vi "FGV_UE.vi"(7 "State":T1, 8 "Error In":errorcluster) -> (0 "Error Out":errorcluster, 3 "STOP":refnum<user-event>)   [LabVIEW 2017, in "StopUE.lvlib"]
uses:
  StopUE.lvlib
  States_FGV.ctl
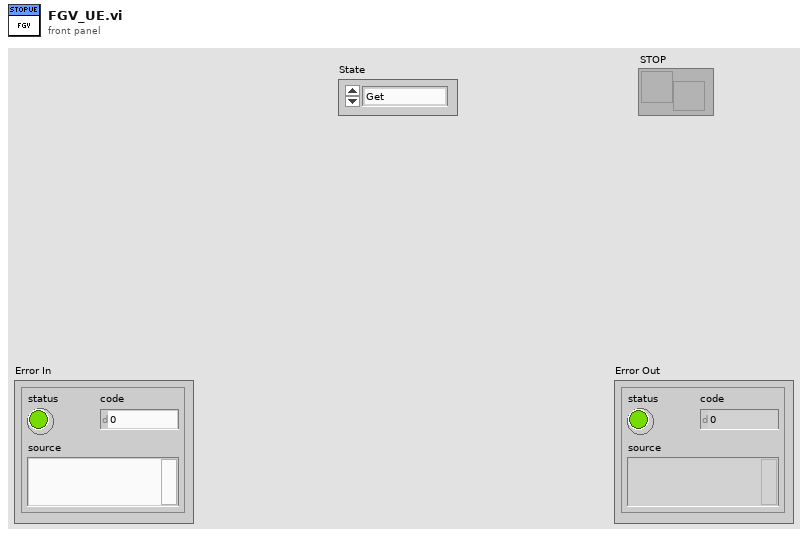
[diagram p1: front panel]
types:
  T1 = typedef "StopUE.lvlib/States_FGV.ctl" = enum16{"Get", "Shutdown", "Initialize"}
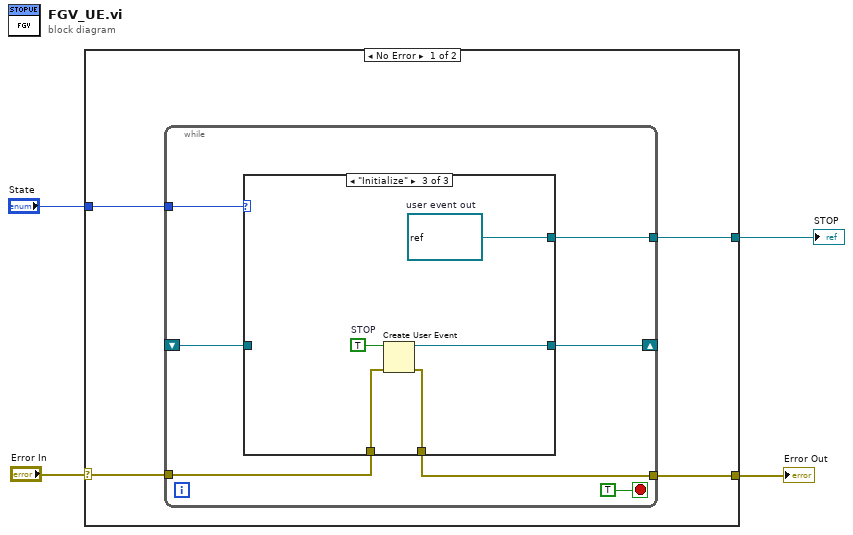
[diagram p0: block diagram]
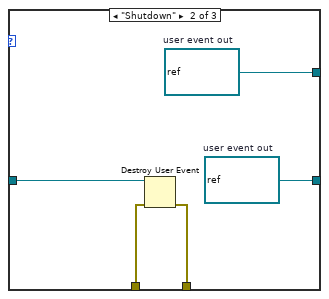
[diagram p3: hidden frame]
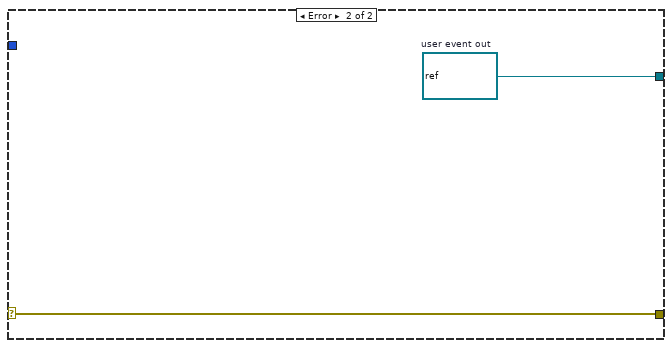
[diagram p4: hidden frame]
diagram:
  n1 = case shown="No Error" "Error In" {
    selector: "Error In" -> [w8 w28]
    tunnel: "State" -> [w7 _]
    tunnel: [w6 w28] -> w2
    tunnel: [w5 w29] -> w1
    frame No Error {
      n2 = while {
        tunnel: w8 -> [w13]
        tunnel: w7 -> [w14]
        tunnel: [w12] -> w6
        shift-right: [w11] -> _
        shift-left: _ -> [w10]
        tunnel: [w9] -> w5
        stop <- TRUE stop-if-true
        n3 = case shown="\"Initialize\"" w14 {
          tunnel: w13 -> [w16 w21 w26]
          tunnel: [w16 w20 w25] -> w12
          tunnel: [w17 w19 w24] -> w11
          tunnel: w10 -> [w17 w22 _]
          tunnel: [w17 w18 w23] -> w9
          frame "Get", Default {
          }
          frame "Shutdown" {
            w18 = refnum<user-event> refnum  # user event out
            w19 = refnum<user-event> refnum  # user event out
            n4 = Destroy User Event(user event=w22, error in=w21) -> (error out=w20:errorcluster)
          }
          frame "Initialize" {
            w23 = refnum<user-event> refnum  # user event out
            w27 = TRUE  # STOP
            n5 = Create User Event(user event datatype=w27, error in=w26) -> (user event=w24:refnum<user-event>, error out=w25:errorcluster)
          }
        }
      }
    }
    frame Error {
      w29 = refnum<user-event> refnum  # user event out
    }
  }
  "Error Out" <- w2
  "STOP" <- w1
